vi "AlazarConfigureRecordAverage.vi"(0 "Handle":u64, 1 "Mode":u32(ring) items=["Disable", "Enable"], 2 "Samples Per Record":u32, 3 "Records Per Average":u32, 4 "Options":u16(ring) items=["Unsigned", "Signed"], 5 "error in (no error)":errorcluster) -> (14 "Handle":u64, 18 "Return Code":u32, 19 "error out":errorcluster)   [LabVIEW 2009]
doc: "This function configures a digitizer to co-add ADC samples from a specified number of records in an accumulator record, and transfer accumulator records rather than the ADC sample values."
uses:
  ATSApi.dll
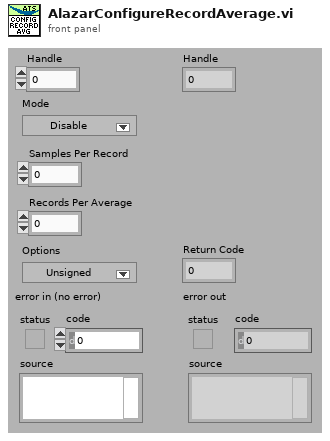
[diagram p1: front panel]
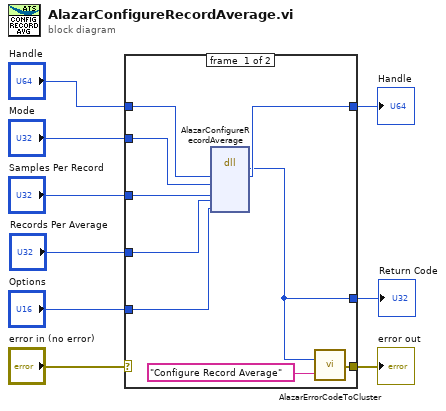
[diagram p0: block diagram]
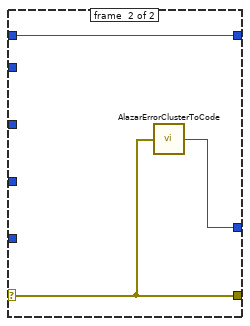
[diagram p2: hidden frame]
diagram:
  n1 = case shown="No Error" "error in (no error)" {
    selector: "error in (no error)" -> [_ w21]
    tunnel: [w12 w21] -> w8
    tunnel: [w11 w20] -> w7
    tunnel: "Handle" -> [w18 w19]
    tunnel: [w17 w19] -> w5
    tunnel: "Mode" -> [w16 _]
    tunnel: "Samples Per Record" -> [w15 _]
    tunnel: "Records Per Average" -> [w14 _]
    tunnel: "Options" -> [w13 _]
    frame #0 {
      n2 = dll-call lib="ATSApi.dll" fn="AlazarConfigureRecordAverage"("handle"=w18, "mode"=w16, "samplesPerRecord"=w15, "recordsPerAverage"=w14, "options"=w13) -> ("return type"=w11:u32, "handle"=w17:u64)  [unwired: 7 in, 2 out]
      n3 = call "AlazarErrorCodeToCluster.vi"("Message"="Configure Record Average", "Error Code"=w11) -> ("error out"=w12:errorcluster)
    }
    frame #1 {
      n4 = call "AlazarErrorClusterToCode.vi"("error in (no error)"=w21) -> ("Error Code"=w20:u32)
    }
  }
  "Handle" <- w5
  "error out" <- w8
  "Return Code" <- w7
